vi "ReadFullMessages.vi"(6 "Timeout(ms)":i32, 8 "error in (no error)":errorcluster, 11 "NetworkConnection in":refnum<class "NetworkConnection.lvclass">) -> (0 "error out":errorcluster, 1 "Messages":T1[](array[typedef]), 2 "StillConnected?":bool, 3 "NetworkConnection out":refnum<class "NetworkConnection.lvclass">, 4 "Timed Out?":bool)   [LabVIEW 2023, in "NetworkConnection.lvclass"]
doc: "Reads all available messages from the Remote System on the Network Connection for the desired timeout period. The messages contain ALL the data including timestamp and other private configuration parameters.\n\nJKI Network Streams Connection 1.1.1.15\nJavier Ruiz - JKI\nCopyright (c) 2020, JKI\n\nThis library is provided \"AS IS\" ,WITHOUT WARRANTIES OR CONDITIONS OF ANY KIND, either express or implied."
uses:
  NetworkConnection.lvclass
  NetworkMessage.ctl
  NetworkCommand.ctl
  NetworkConnection.lvclass/NetworkConnection.ctl
  <resource>/objmgr/ni.dex.rc
panel:
  # "Copyright © 2020 JKI All rights reserved.\n\nAuthor: Javier Ruiz <javier.ruiz@jki.net>\n\nThis library is provided \"AS IS\" ,WITHOUT WARRANTIES OR \nCONDITIONS OF ANY KIND, either expressed or implied.\n\nJKI -- jki.net"
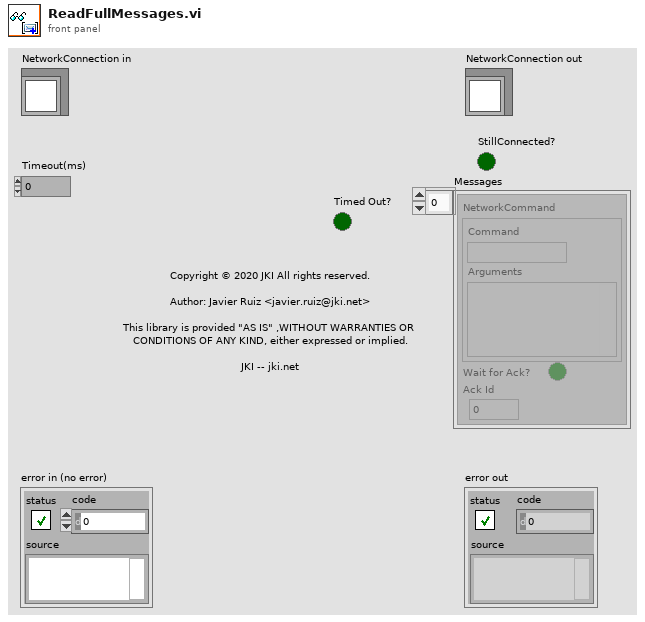
[diagram p1: front panel]
types:
  T1 = typedef "NetworkConnection.lvclass/NetworkMessage.ctl" = cluster{"NetworkCommand":T2, "Wait for Ack?":bool, "Ack Id":i32}
  T2 = typedef "NetworkConnection.lvclass/NetworkCommand.ctl" = cluster{"Command":string, "Arguments":variant}
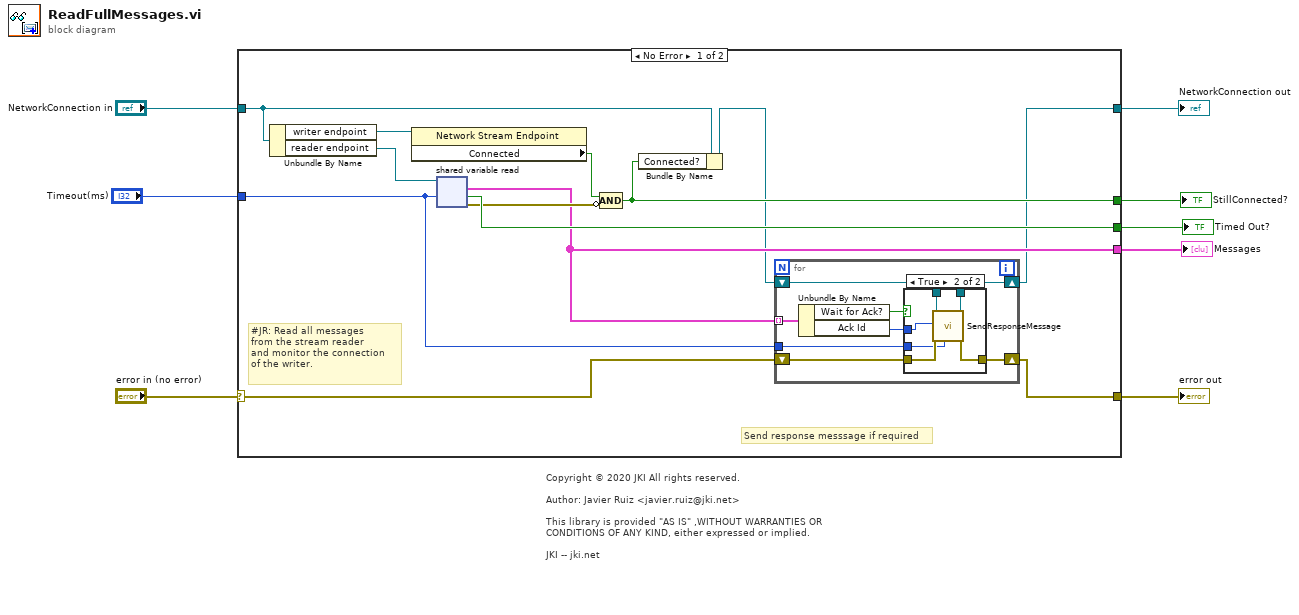
[diagram p0: block diagram]
diagram:
  # "Copyright © 2020 JKI All rights reserved.\n\nAuthor: Javier Ruiz <javier.ruiz@jki.net>\n\nThis library is provided \"AS IS\" ,WITHOUT WARRANTIES OR \nCONDITIONS OF ANY KIND, either expressed or implied.\n\nJKI -- jki.net"
  n1 = case shown="No Error" "error in (no error)" {
    selector: "error in (no error)" -> [w13 w39]
    tunnel: [w12 w39] -> w7
    tunnel: [w9 w38] -> w5
    tunnel: "NetworkConnection in" -> [w18 w38]
    tunnel: "Timeout(ms)" -> [w11 _]
    tunnel: [w14 _] -> w3
    tunnel: [w17 _] -> w2
    tunnel: [w19 _] -> w1
    frame No Error {
      # "Send response messsage if required"
      # "#JR: Read all messages\nfrom the stream reader\nand monitor the connection\nof the writer."
      n2 = Unbundle By Name(w18) -> ("writer endpoint"=w20:refnum<k21>, "reader endpoint"=w21:refnum<k21>)
      n3 = property class="Network Stream Endpoint"(reference=w20) -> ("Connected"=w16:bool)  [unwired: 1 in, 2 out]
      n4 = shared-variable-read(w21, w11) -> (w15:errorcluster, w19:bool, w14:T1[])  [unwired: 2 in, 1 out]
      n5 = Compound Arithmetic op=AND(w16, invert w15) -> (w17:bool)
      n6 = Bundle By Name(cluster=w18, "Connected?"=w17) -> (w10:refnum<class "NetworkConnection.lvclass">)
      n7 = for {
        tunnel: w14 -> [w29] mode=indexing
        shift-right: [w26] -> w12
        shift-left: w13 -> [w27]
        tunnel: w11 -> [w24]
        shift-right: [w22] -> w9
        shift-left: w10 -> [w23]
        n8 = Unbundle By Name(w29) -> ("Wait for Ack?"=w28:bool, "Ack Id"=w25:i32)
        n9 = case shown="True" w28 {
          tunnel: w23 -> [w30 w37]
          tunnel: [w30 w36] -> w22
          tunnel: w27 -> [w31 w34]
          tunnel: [w31 w35] -> w26
          tunnel: w25 -> [_ w33]
          tunnel: w24 -> [_ w32]
          frame False {
          }
          frame True {
            n10 = call "SendResponseMessage.vi"("Timeout(ms)"=w32, "error in (no error)"=w34, "Ack Id"=w33, "NetworkConnection in"=w37) -> ("error out"=w35:errorcluster, "NetworkConnection out"=w36:refnum<class "NetworkConnection.lvclass">)  [unwired: 4 in, 2 out]
          }
        }
      }
    }
    frame Error {
    }
  }
  "error out" <- w7
  "NetworkConnection out" <- w5
  "StillConnected?" <- w2
  "Messages" <- w3
  "Timed Out?" <- w1
